vi "电压采样检测.vi"(0 "仪器实例 in":T1, 11 "error in (no error)":errorcluster) -> (3 "全部打开":T2, 4 "闭合主正":T2, 6 "闭合主正快充":T2, 10 "短接快充":T2, 13 "表格控件":string[][](table) caption="电压采样精度检测", 14 "?":bool, 15 "error out":errorcluster caption="错误输出")   [LabVIEW 2020]
uses:
  F:/F020/S7_1200 control/HslCommunication.dll
  S7_1200 control/HslCommunication.dll
  S7_1200 control/S7_1200 WriteBools.vi
  S7_1200 control/S7_1200 WriteBool.vi
  <instrlib>/Keithley 24XX/Public/Data/Read (Single Point).vi
  <instrlib>/Keithley 24XX/Keithley 24XX.lvlib
  S7_1200 control/S7_1200 control.lvlib
panel:
  # "F020 电压采样检测"
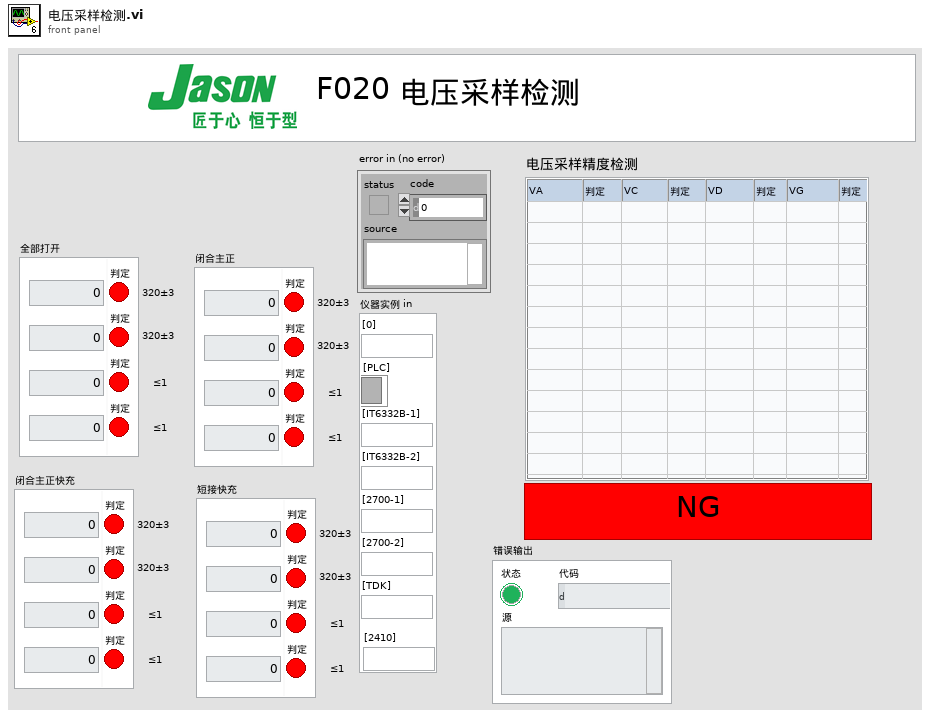
[diagram p1: front panel]
types:
  T1 = typedef "仪器实例.ctl" = cluster{"[0]":string, "[PLC]":refnum<k24>, "[IT6332B-1]":string, "[IT6332B-2]":string, "[2700-1]":string, "[2700-2]":string, "[TDK]":string, "[2410]":string}
  T2 = typedef "闭合主正.ctl" = cluster{"簇":cluster{"Va":u32, "Vc":u32, "Vd":u32, "Vg":u32}, "判定":cluster{"判定":bool, "判定":bool, "判定":bool, "判定":bool}}
  T3 = cluster{"电压[0]":u32, "电压[1]":u32, "电压[2]":u32, "电压[3]":u32}
  T4 = cluster{"判定结果数组[0]":bool, "判定结果数组[1]":bool, "判定结果数组[2]":bool, "判定结果数组[3]":bool}
  T5 = cluster{"电压":cluster{"电压[0]":u32, "电压[1]":u32, "电压[2]":u32, "电压[3]":u32}, "判定结果数组":cluster{"判定结果数组[0]":bool, "判定结果数组[1]":bool, "判定结果数组[2]":bool, "判定结果数组[3]":bool}}
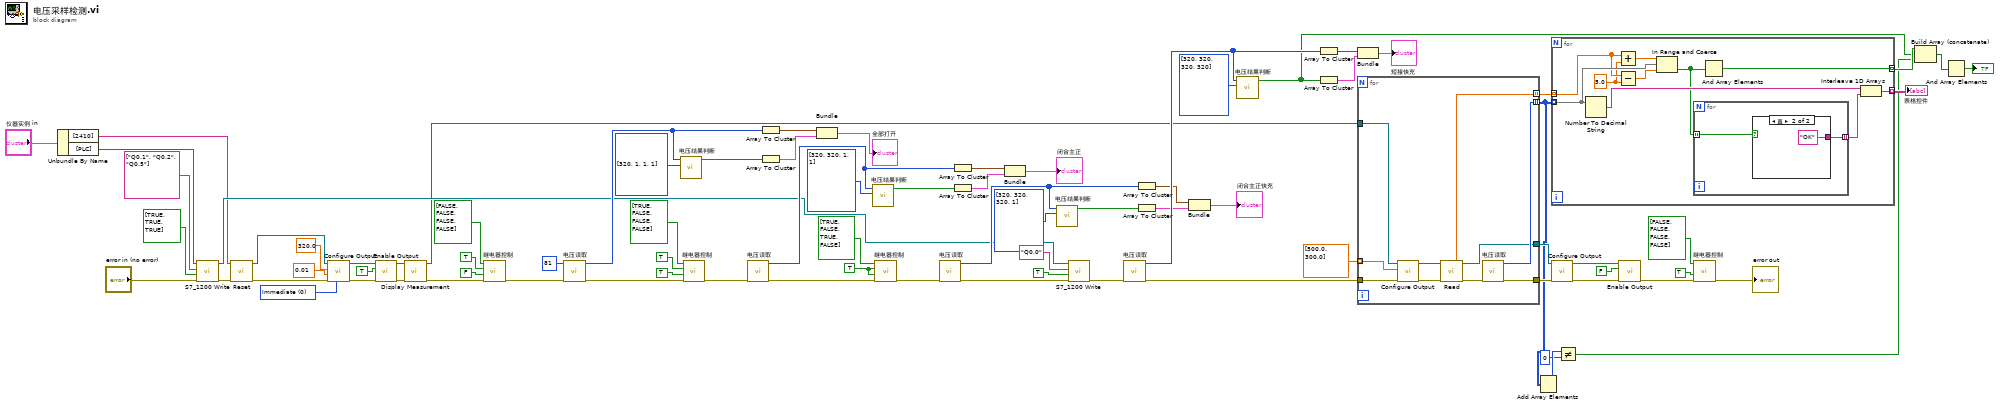
[diagram p0: block diagram]
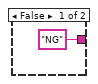
[diagram p2: hidden frame]
diagram:
  w23 = TRUE ("释放")
  w80 = u16 0 items=["Immediate", "Triggered"] ("Output Type  (0: Immediate)")
  n1 = Unbundle By Name("仪器实例 in") -> ("[2410]"=w20:string, "[PLC]"=w21:refnum<k24>)
  n2 = call-poly "S7_1200 Write.vi"("错误输入（无错误）"="error in (no error)", "values"=bool[] [TRUE, TRUE, TRUE], "addresses"=string[] ["Q0.1", "Q0.2", "Q0.5"], "引用"=w21) -> ("错误输出"=w28:errorcluster, "引用输出"=w36:refnum<k24>)  [unwired: 2 in]
  n3 = call <instrlib>:"Reset.vi"("error in (no error)"=w28, "VISA resource name"=w20) -> ("error out"=w27:errorcluster, "VISA resource name out"=w29:refnum<visa-resource-name>)  [unwired: 8 in]
  n4 = call <instrlib>:"Configure Output.vi"("Output Type  (0: Immediate)"=w80, "error in (no error)"=w27, "Compliance  Level (0.1)"=0.01, "Output Level (0)"=320.0, "VISA resource name"=w29) -> ("error out"=w79:errorcluster, "VISA resource name out"=w78:refnum<visa-resource-name>)  [unwired: 5 in]
  n5 = call <instrlib>:"Enable Output.vi"("error in (no error)"=w79, "Enable Output (T: Enable)"=TRUE, "VISA resource name"=w78) -> ("error out"=w32:errorcluster, "VISA resource name out"=w33:refnum<visa-resource-name>)  [unwired: 7 in]
  n6 = call <instrlib>:"Display Measurement.vi"("error in (no error)"=w32, "VISA resource name"=w33) -> ("error out"=w31:errorcluster, "VISA resource name out"=w30:refnum<visa-resource-name>)  [unwired: 8 in]
  n7 = call "继电器控制.vi"("error in"=w31, "释放"=FALSE, "初始化"=TRUE, "继电器控制"=bool[] [FALSE, FALSE, FALSE, FALSE]) -> ("error out"=w60:errorcluster)  [unwired: 7 in]
  n8 = call "电压读取.vi"("error in"=w60, "Channel"=u16 81) -> ("error out"=w76:errorcluster, "电压"=w54:u32[])  [unwired: 8 in]
  n9 = call "电压结果判断.vi"("判定阈值"=u32[] [320, 1, 1, 1], "电压数组"=w54) -> ("判定结果数组"=w44:bool[])  [unwired: 6 in, 1 out]
  n10 = call "继电器控制.vi"("error in"=w76, "释放"=TRUE, "初始化"=TRUE, "继电器控制"=bool[] [TRUE, FALSE, FALSE, FALSE]) -> ("error out"=w74:errorcluster)  [unwired: 7 in]
  n11 = call "电压读取.vi"("error in"=w74) -> ("error out"=w73:errorcluster, "电压"=w52:u32[])  [unwired: 9 in]
  n12 = Array To Cluster(array=w54) -> (cluster=w42:T3)
  n13 = Array To Cluster(array=w44) -> (cluster=w43:T4)
  n14 = Bundle("电压"=w42, "判定结果数组"=w43) -> (→"全部打开":T5)  [unwired: 1 in]
  n15 = call "电压结果判断.vi"("判定阈值"=u32[] [320, 320, 1, 1], "电压数组"=w52) -> ("判定结果数组"=w41:bool[])  [unwired: 6 in, 1 out]
  n16 = call "继电器控制.vi"("error in"=w73, "释放"=w23, "初始化"=w23, "继电器控制"=bool[] [TRUE, FALSE, TRUE, FALSE]) -> ("error out"=w71:errorcluster)  [unwired: 7 in]
  n17 = call "电压读取.vi"("error in"=w71) -> ("error out"=w58:errorcluster, "电压"=w50:u32[])  [unwired: 9 in]
  n18 = Array To Cluster(array=w52) -> (cluster=w17:T3)
  n19 = Array To Cluster(array=w41) -> (cluster=w16:T4)
  n20 = Bundle("电压"=w17, "判定结果数组"=w16) -> (→"闭合主正":T5)  [unwired: 1 in]
  n21 = call "电压结果判断.vi"("判定阈值"=u32[] [320, 320, 320, 1], "电压数组"=w50) -> ("判定结果数组"=w40:bool[])  [unwired: 6 in, 1 out]
  n22 = call-poly "S7_1200 Write.vi"("错误输入（无错误）"=w58, "value"=TRUE, "address"="Q0.0", "引用"=w36) -> ("错误输出"=w55:errorcluster)  [unwired: 2 in, 1 out]
  n23 = call "电压读取.vi"("error in"=w55) -> ("error out"=w8:errorcluster, "电压"=w47:u32[])  [unwired: 9 in]
  n24 = Array To Cluster(array=w50) -> (cluster=w13:T3)
  n25 = Array To Cluster(array=w40) -> (cluster=w12:T4)
  n26 = Bundle("电压"=w13, "判定结果数组"=w12) -> (→"闭合主正快充":T5)  [unwired: 1 in]
  n27 = call "电压结果判断.vi"("判定阈值"=u32[] [320, 320, 320, 320], "电压数组"=w47) -> ("判定结果数组"=w6:bool[])  [unwired: 6 in, 1 out]
  n28 = Array To Cluster(array=w47) -> (cluster=w11:T3)
  n29 = Array To Cluster(array=w6) -> (cluster=w10:T4)
  n30 = Bundle("电压"=w11, "判定结果数组"=w10) -> (→"短接快充":T5)  [unwired: 1 in]
  n31 = for {
    tunnel: dbl[] [500.0, 300.0] -> [w92] mode=indexing
    tunnel: w30 -> [w91]
    tunnel: [w90] -> w69
    tunnel: [w84] -> w68
    tunnel: [w89] -> w3 mode=indexing
    tunnel: w8 -> [w88]
    tunnel: [w83] -> w63 mode=indexing
    n32 = call <instrlib>:"Configure Output.vi"("error in (no error)"=w88, "Output Level (0)"=w92, "VISA resource name"=w91) -> ("error out"=w87:errorcluster, "VISA resource name out"=w85:refnum<visa-resource-name>)  [unwired: 7 in]
    n33 = call-poly <instrlib>:"Read.vi"("VISA resource name"=w85, "error in (no error)"=w87) -> ("Voltage"=w83:sgl, "VISA resource name out"=w84:refnum<visa-resource-name>, "error out"=w86:errorcluster)  [unwired: 7 in, 4 out]
    n34 = call "电压读取.vi"("error in"=w86) -> ("error out"=w90:errorcluster, "电压"=w89:u32[])  [unwired: 9 in]
  }
  n35 = Add Array Elements(numeric array=w3) -> (sum=w2:u32)
  n36 = for {
    tunnel: w3 -> [w100] mode=indexing
    tunnel: w63 -> [w94] mode=indexing
    tunnel: [w97] -> w61 mode=indexing
    tunnel: [w95] -> w7 mode=indexing
    w93 = sgl 5.0 ("y")
    n37 = Number To Decimal String(number=w100) -> (decimal integer string=w99:string[])  [unwired: 1 in]
    n38 = Add(x=w94, y=w93) -> (x+y=w102:sgl)
    n39 = Subtract(x=w94, y=w93) -> (x-y=w101:sgl)
    n40 = In Range and Coerce(upper limit=w102, x=w100, lower limit=w101) -> (In Range?=w96:bool[])  [unwired: 1 out]
    n41 = for {
      tunnel: w96 -> [w104] mode=indexing
      tunnel: [w103] -> w98 mode=indexing
      n42 = case shown="真" w104 {
        tunnel: ["NG" "OK"] -> w103
        frame False {
        }
        frame True {
        }
      }
    }
    n43 = And Array Elements(Boolean array=w96) -> (logical AND=w95:bool)
    n44 = Interleave 1D Arrays(w99, w98) -> (w97:string[])
  }
  "表格控件" <- w61
  n45 = call <instrlib>:"Configure Output.vi"("error in (no error)"=w69, "VISA resource name"=w68) -> ("error out"=w67:errorcluster, "VISA resource name out"=w66:refnum<visa-resource-name>)  [unwired: 8 in]
  n46 = Not Equal?(x=w2, y=u32 0) -> (x != y?=w4:bool)
  n47 = call <instrlib>:"Enable Output.vi"("error in (no error)"=w67, "Enable Output (T: Enable)"=FALSE, "VISA resource name"=w66) -> ("error out"=w35:errorcluster)  [unwired: 7 in, 1 out]
  n48 = call "继电器控制.vi"("error in"=w35, "释放"=TRUE, "继电器控制"=bool[] [FALSE, FALSE, FALSE, FALSE]) -> ("error out"=→"error out":errorcluster)  [unwired: 8 in]
  n49 = Build Array (concatenate)(w7, w6, w4) -> (w5:bool[])
  n50 = And Array Elements(Boolean array=w5) -> (logical AND=→"?":bool)
